vi "Measure.vi"(8 "error in (no error)":errorcluster, 9 "measurement configuration":variant, 10 "measure call context in":refnum<class "Measure Call Context.lvclass">, 11 "measurement plugin in":refnum<class "FPT_SParam.lvclass">) -> (0 "error out":errorcluster, 1 "measurement results":variant, 2 "measure call context out":refnum<class "Measure Call Context.lvclass">, 3 "measurement plugin out":refnum<class "FPT_SParam.lvclass">)   [LabVIEW 2023, in "FPT_SParam.lvclass"]
uses:
  FPT_SParam.lvclass
  <vilib>/Plug-In SDKs/Measurements/Measure Call Context/Measure Call Context.lvclass
  Measurement Configuration.ctl
  FPT_SParam.lvclass/FPT_SParam.ctl
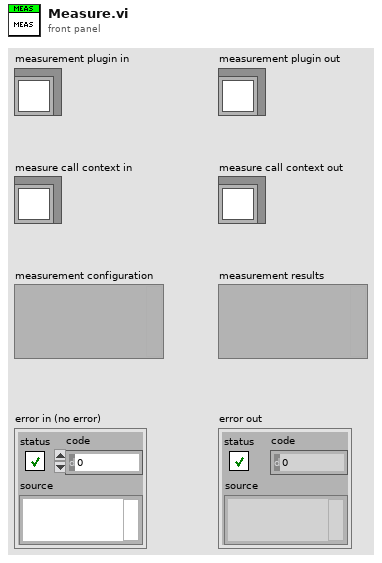
[diagram p1: front panel]
types:
  T1 = typedef "FPT_SParam.lvclass/Measurement Configuration.ctl" = cluster{"Automation Test":bool, "Power sequencing file path":string, "RFmxVNA name":string, "vCal Name":string, "RFmxVNA Calset Enable":bool, "RFmxVNA Calset Interpolation":bool, "Calset File Path (String)":string, "RFmxVNA attenuation mode":enum32{"<None>", "s2p File"}, "RFmxVNA Port1 s2p file path (String)":string, "RFmxVNA Port1 s-parameters orientation":enum32{"Port1 Towards DUT", "Port2 Towards DUT"}, "RFmxVNA Port1 Power Compensation":bool, "RFmxVNA Port2 s2p file path (String)":string, "RFmxVNA Port2 s-parameters orientation":enum32{"Port1 Towards DUT", "Port2 Towards DUT"}, "RFmxVNA Port2 Power Compensation":bool, "Port1 Power Level (dBm)":dbl, "Port1 Test Receiver Attenuation (dB)":dbl, "Port2 Power Level (dBm)":dbl, "Port2 Test Receiver Attenuation (dB)":dbl, "IF Bandwidth (Hz)":dbl, "Action":enum32{"Calibrate", "Measure"}, "Pulse Mode Enabled":bool, "Pulse Period":dbl, "Pulse Modulator Delay":dbl, "Pulse Modulator Width":dbl, "Pulse Acquisition Auto":bool, "Pulse Acquisition Delay":dbl, "Pulse Acquisition Width":dbl, "Start Frequency (Hz)":dbl, "Stop Frequency (Hz)":dbl, "Number of Points":i32, "Measurement S-Parameters":string[], "Phase Trace Type":i32, "Magnitude Units":i32, "SnP File Path (String)":string, "Averaging Enabled":bool, "Averaging Count":u32, "Power sequencing file validity check":bool}
  T2 = typedef "FPT_SParam.lvclass/Measurement Results.ctl" = cluster{"Status":string, "S-Param Name":string[], "S-Param Magnitude":dbl[][], "S-Param Phase":dbl[][], "S21 (Mean)":dbl, "S12 (Mean)":dbl, "VNA Status":string}
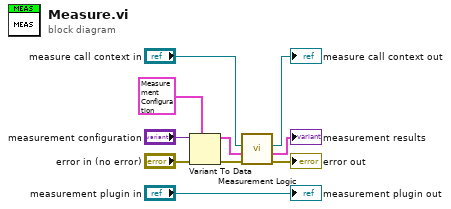
[diagram p0: block diagram]
diagram:
  n1 = Variant To Data(error in="error in (no error)", type=T1 {"Automation Test"=FALSE, "Power sequencing file path"="Lorem ipsum dolor sit", "RFmxVNA name"="5842_0", "vCal Name"="", "RFmxVNA Calset Enable"=FALSE, "RFmxVNA Calset Interpolation"=FALSE, "Calset File Path (String)"="", "RFmxVNA attenuation mode"=enum."s2p File", "RFmxVNA Port1 s2p file path (String)"="", "RFmxVNA Port1 s-parameters orientation"=enum."Port1 Towards DUT", "RFmxVNA Port1 Power Compensation"=FALSE, "RFmxVNA Port2 s2p file path (String)"="", "RFmxVNA Port2 s-parameters orientation"=enum."Port1 Towards DUT", "RFmxVNA Port2 Power Compensation"=FALSE, "Port1 Power Level (dBm)"=1.0, "Port1 Test Receiver Attenuation (dB)"=1.0, "Port2 Power Level (dBm)"=1.0, "Port2 Test Receiver Attenuation (dB)"=1.0, "IF Bandwidth (Hz)"=1.0, "Action"=enum."Measure", "Pulse Mode Enabled"=FALSE, "Pulse Period"=0.001, "Pulse Modulator Delay"=0.0, "Pulse Modulator Width"=0.0001, "Pulse Acquisition Auto"=FALSE, "Pulse Acquisition Delay"=2e-05, "Pulse Acquisition Width"=4.665e-05, "Start Frequency (Hz)"=4000000000.0, "Stop Frequency (Hz)"=26000000000.0, "Number of Points"=200, "Measurement S-Parameters"=["S11", "S12", "S21", "S22"], "Phase Trace Type"=0, "Magnitude Units"=0, "SnP File Path (String)"="", "Averaging Enabled"=FALSE, "Averaging Count"=0, "Power sequencing file validity check"=TRUE} ("measurement configuration"), Variant="measurement configuration") -> (data=w1:T1, error out=w7:errorcluster)
  n2 = call "Measurement Logic.vi"("error in"=w7, "measurement configuration"=w1, "measure call context in"="measure call context in") -> ("error out"=→"error out":errorcluster, "measurement results"=→"measurement results":T2, "measure call context out"=→"measure call context out":refnum<class "Measure Call Context.lvclass">)  [unwired: 6 in]
  "measurement plugin out" <- "measurement plugin in"
